vi "Calibration-Fit-(SubVI).vi"(10 "Array in":dbl[][](array[numeric])) -> (1 "intercept":dbl, 2 "slope":dbl, 3 "Array out":cluster{dbl[], "Best Linear Fit":dbl[]}[](array[cluster]), 4 "Array 3":dbl[](array[numeric])=[1.0, 2.0, 3.0, 4.0, 5.0])   [LabVIEW 2024]
uses:
  <vilib>/Analysis/NI_AALPro.lvlib
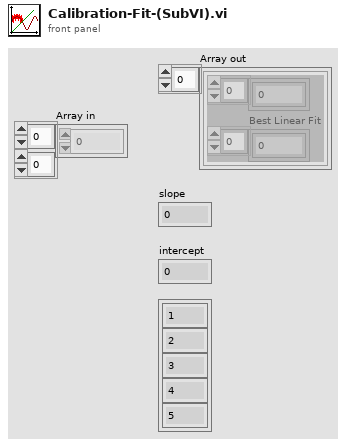
[diagram p1: front panel]
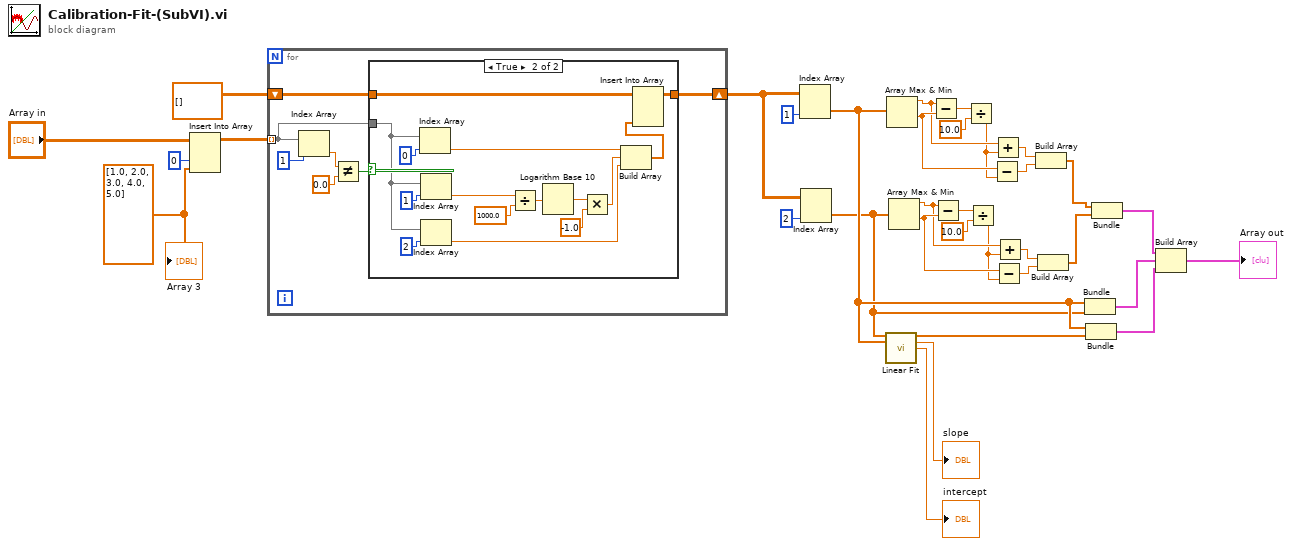
[diagram p0: block diagram]
diagram:
  w31 = dbl[] [1.0, 2.0, 3.0, 4.0, 5.0]
  n1 = Insert Into Array(array="Array in", index (col)=0 ("disabled index (col)"), new element=w31) -> (w6:dbl[][])  [unwired: 1 in]
  n2 = for {
    tunnel: w6 -> [w36] mode=indexing
    shift-right: [w35] -> w26
    shift-left: dbl[][] [] -> [w37]
    n3 = Index Array(array=w36, index=1) -> (element=w39:dbl)
    n4 = Not Equal?(x=w39, y=0.0) -> (x != y?=w34:bool)
    n5 = case shown="True" w34 {
      tunnel: w37 -> [w41 w56]
      tunnel: w36 -> [_ w51]
      tunnel: [w41 w55] -> w35
      frame False {
      }
      frame True {
        n6 = Index Array(array=w51, index=0) -> (element=w46:dbl)
        n7 = Index Array(array=w51, index=1) -> (element=w42:dbl)
        n8 = Index Array(array=w51, index=2) -> (element=w47:dbl)
        n9 = Divide(x=w42, y=1000.0) -> (x/y=w44:dbl)
        n10 = Logarithm Base 10(1:w44) -> (0:w50:dbl)
        n11 = Multiply(x=w50, y=-1.0) -> (x*y=w48:dbl)
        n12 = Build Array(w46, w48, w47) -> (w45:dbl[])
        n13 = Insert Into Array(array=w56, new element=w45) -> (w55:dbl[][])  [unwired: 2 in]
      }
    }
  }
  n14 = Index Array(array=w26, index (col)=1 ("disabled index (col)")) -> (element=w28:dbl[])  [unwired: 1 in]
  n15 = Index Array(array=w26, index (col)=2 ("disabled index (col)")) -> (element=w27:dbl[])  [unwired: 1 in]
  n16 = call <vilib>:"Linear Fit.vi"("Y"=w27, "X"=w28) -> ("Best Linear Fit"=w29:dbl[], "slope"=→"slope":dbl, "intercept"=→"intercept":dbl)  [unwired: 9 in, 2 out]
  n17 = Array Max & Min(array=w28) -> (max value=w10:dbl, min value=w11:dbl)  [unwired: 2 out]
  n18 = Array Max & Min(array=w27) -> (max value=w17:dbl, min value=w18:dbl)  [unwired: 2 out]
  n19 = Subtract(x=w10, y=w11) -> (x-y=w7:dbl)
  n20 = Subtract(x=w17, y=w18) -> (x-y=w14:dbl)
  n21 = Divide(x=w7, y=10.0) -> (x/y=w9:dbl)
  n22 = Divide(x=w14, y=10.0) -> (x/y=w16:dbl)
  n23 = Subtract(x=w11, y=w9) -> (x-y=w13:dbl)
  n24 = Add(x=w10, y=w9) -> (x+y=w12:dbl)
  n25 = Subtract(x=w18, y=w16) -> (x-y=w20:dbl)
  n26 = Add(x=w17, y=w16) -> (x+y=w19:dbl)
  n27 = Build Array(w12, w13) -> (w21:dbl[])
  n28 = Build Array(w19, w20) -> (w22:dbl[])
  n29 = Bundle(w28, w27) -> (w24:cluster{dbl[], dbl[]})  [unwired: 1 in]
  n30 = Bundle(w28, "Best Linear Fit"=w29) -> (w30:cluster{dbl[], "Best Linear Fit":dbl[]})  [unwired: 1 in]
  n31 = Bundle(w21, w22) -> (w23:cluster{dbl[], dbl[]})  [unwired: 1 in]
  n32 = Build Array(w23, w24, w30) -> (→"Array out":cluster{dbl[], "Best Linear Fit":dbl[]}[])
  "Array 3" <- w31
